vi "Section to Variant Attributes.vi"(8 "error in":errorcluster, 9 "section":string, 10 "variant in":variant, 11 "Refnum in":T1) -> (0 "error out":errorcluster, 2 "variant out":variant, 3 "Refnum out":T1)   [LabVIEW 2014]
uses:
  <vilib>/Utility/config.llb/Config Data RefNum.ctl
  <vilib>/Utility/config.llb/Read Key (I32).vi
  <vilib>/Utility/config.llb/Read Key (Double).vi
  <vilib>/Utility/config.llb/Read Key (String).vi
  <vilib>/Utility/config.llb/Read Key (Path).vi
  <vilib>/Utility/config.llb/Read Key (Boolean).vi
  <vilib>/Utility/config.llb/NI_LVConfig.lvlib
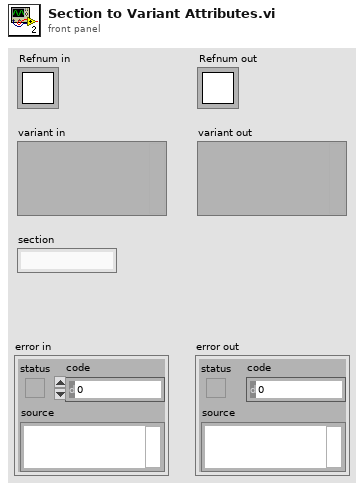
[diagram p1: front panel]
types:
  T1 = typedef "NI_LVConfig.lvlib/Config Data RefNum.ctl" = refnum<k1>
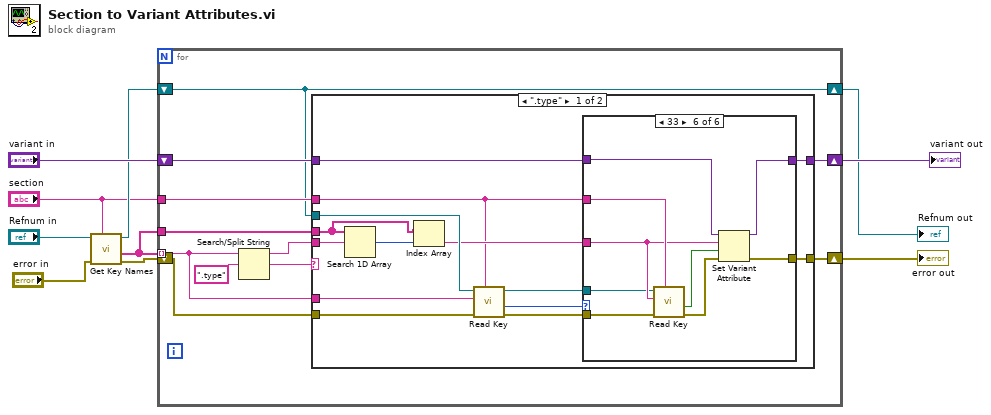
[diagram p0: block diagram]
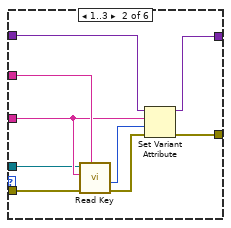
[diagram p3: hidden frame]
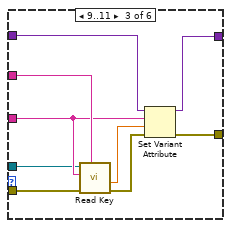
[diagram p4: hidden frame]
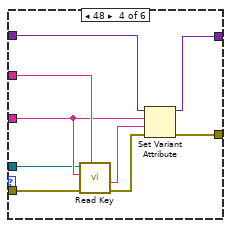
[diagram p5: hidden frame]
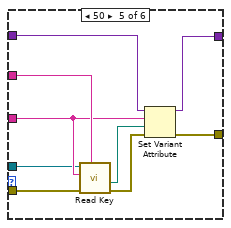
[diagram p6: hidden frame]
diagram:
  n1 = call <vilib>:"Get Key Names.vi"("section"="section", "error in (no error)"="error in", "refnum"="Refnum in") -> ("error out"=w8:errorcluster, "key names"=w3:string[], "refnum out"=w5:T1)  [unwired: 5 in, 1 out]
  n2 = for {
    tunnel: w3 -> [w16] mode=indexing
    tunnel: w3 -> [w18]
    tunnel: "section" -> [w17]
    shift-right: [w14] -> w10
    shift-left: "variant in" -> [w15]
    shift-right: [w13] -> w7
    shift-left: w5 -> [w13]
    shift-right: [w11] -> w9
    shift-left: w8 -> [w12]
    n3 = Search/Split String(string=w16, search string/char (-)=".type") -> (substring before match=w19:string, match + rest of string=w20:string)  [unwired: 1 in, 1 out]
    n4 = case shown="\".type\"" w20 {
      tunnel: w19 -> [w35 _]
      tunnel: w18 -> [w34 _]
      tunnel: w17 -> [w26 _]
      tunnel: w13 -> [w32 _]
      tunnel: w16 -> [w31 _]
      tunnel: w15 -> [w30 w84]
      tunnel: [w28 w84] -> w14
      tunnel: w12 -> [w24 w83]
      tunnel: [w23 w83] -> w11
      frame ".type" {
        n5 = Search 1D Array(1D array=w34, element=w35) -> (index of element=w33:i32)  [unwired: 1 in]
        n6 = Index Array(array=w34, index=w33) -> (element=w29:string)
        n7 = call-poly <vilib>:"Read Key.vi"("section"=w26, "error in (no error)"=w24, "key"=w31, "refnum"=w32) -> ("error out"=w27:errorcluster, "value"=w22:i32, "refnum out"=w25:T1)  [unwired: 4 in, 1 out]
        n8 = case shown="33" w22 {
          tunnel: w30 -> [w37 w46 w55 w64 w73 w82]
          tunnel: w29 -> [_ w40 w49 w58 w67 w76]
          tunnel: [w37 w45 w54 w63 w72 w81] -> w28
          tunnel: w27 -> [w36 w42 w51 w60 w69 w78]
          tunnel: w26 -> [_ w41 w50 w59 w68 w77]
          tunnel: w25 -> [_ w38 w47 w56 w65 w75]
          tunnel: [w36 w39 w48 w57 w66 w74] -> w23
          frame 0, Default {
          }
          frame 1..3 {
            n9 = call-poly <vilib>:"Read Key.vi"("section"=w41, "error in (no error)"=w42, "key"=w40, "refnum"=w38) -> ("error out"=w43:errorcluster, "value"=w44:i32)  [unwired: 4 in, 2 out]
            n10 = Set Variant Attribute(Variant=w46, name=w40, value=w44, error in=w43) -> (Variant out=w45:variant, error out=w39:errorcluster)  [unwired: 1 out]
          }
          frame 9..11 {
            n11 = call-poly <vilib>:"Read Key.vi"("section"=w50, "error in (no error)"=w51, "key"=w49, "refnum"=w47) -> ("error out"=w52:errorcluster, "value"=w53:dbl)  [unwired: 4 in, 2 out]
            n12 = Set Variant Attribute(Variant=w55, name=w49, value=w53, error in=w52) -> (Variant out=w54:variant, error out=w48:errorcluster)  [unwired: 1 out]
          }
          frame 48 {
            n13 = call-poly <vilib>:"Read Key.vi"("section"=w59, "error in (no error)"=w60, "key"=w58, "refnum"=w56) -> ("error out"=w61:errorcluster, "value"=w62:string)  [unwired: 4 in, 2 out]
            n14 = Set Variant Attribute(Variant=w64, name=w58, value=w62, error in=w61) -> (Variant out=w63:variant, error out=w57:errorcluster)  [unwired: 1 out]
          }
          frame 50 {
            n15 = call-poly <vilib>:"Read Key.vi"("section"=w68, "error in (no error)"=w69, "key"=w67, "refnum"=w65) -> ("error out"=w70:errorcluster, "value"=w71:path)  [unwired: 4 in, 2 out]
            n16 = Set Variant Attribute(Variant=w73, name=w67, value=w71, error in=w70) -> (Variant out=w72:variant, error out=w66:errorcluster)  [unwired: 1 out]
          }
          frame 33 {
            n17 = call-poly <vilib>:"Read Key.vi"("section"=w77, "error in (no error)"=w78, "key"=w76, "refnum"=w75) -> ("error out"=w79:errorcluster, "value"=w80:bool)  [unwired: 4 in, 2 out]
            n18 = Set Variant Attribute(Variant=w82, name=w76, value=w80, error in=w79) -> (Variant out=w81:variant, error out=w74:errorcluster)  [unwired: 1 out]
          }
        }
      }
      frame "True", Default {
      }
    }
  }
  "variant out" <- w10
  "error out" <- w9
  "Refnum out" <- w7
